vi "FiberSpectrograph_monitorCommand_abort.vi"(8 "error in (no error)":errorcluster, 11 "command_abort_Ctl":T1) -> (0 "error out":errorcluster, 2 "function return":i32, 3 "command_abort_Ctl out":T1)   [LabVIEW 2016, in "SALLV_FiberSpectrograph.lvlib"]
doc: "int FiberSpectrograph_shm_monitorCommand_abortLV(FiberSpectrograph_command_abortLV *command_abort_Ctl );"
uses:
  SALLV_FiberSpectrograph.lvlib
  DataTypes/command_abort.ctl
  SALLV_FiberSpectrograph.so
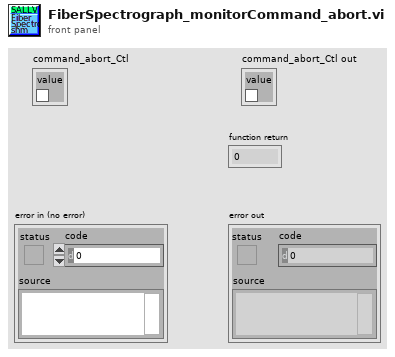
[diagram p1: front panel]
types:
  T1 = typedef "SALLV_FiberSpectrograph.lvlib/command_abort.ctl" = cluster{"value":bool}
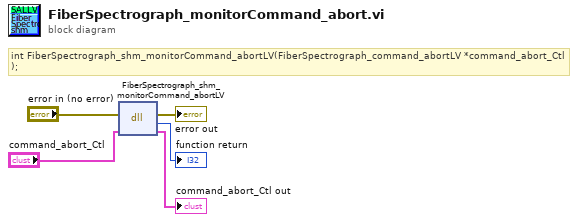
[diagram p0: block diagram]
diagram:
  # "int FiberSpectrograph_shm_monitorCommand_abortLV(FiberSpectrograph_command_abortLV *command_abort_Ctl );"
  n1 = dll-call lib="home/harini/Documents/lsst/SALLV_FiberSpectrograph/SALLV_FiberSpectrograph.*" fn="FiberSpectrograph_shm_monitorCommand_abortLV"(error in="error in (no error)", "command_abort_Ctl"="command_abort_Ctl") -> (error out=→"error out":errorcluster, →"function return":i32, "command_abort_Ctl"=→"command_abort_Ctl out":T1)  [unwired: 2 in, 1 out]
